vi "Write COM Port.vi"(8 "error in (no error)":errorcluster, 10 "COM Port":refnum<visa-resource-name>, 11 "AirMar in":refnum<class "AirMar.lvclass">) -> (0 "error out":errorcluster, 3 "AirMar out":refnum<class "AirMar.lvclass">)   [LabVIEW 2017, in "Sensors.lvlib" / "AirMar.lvclass"]
uses:
  AirMar.lvclass
  AirMar.lvclass/AirMar.ctl
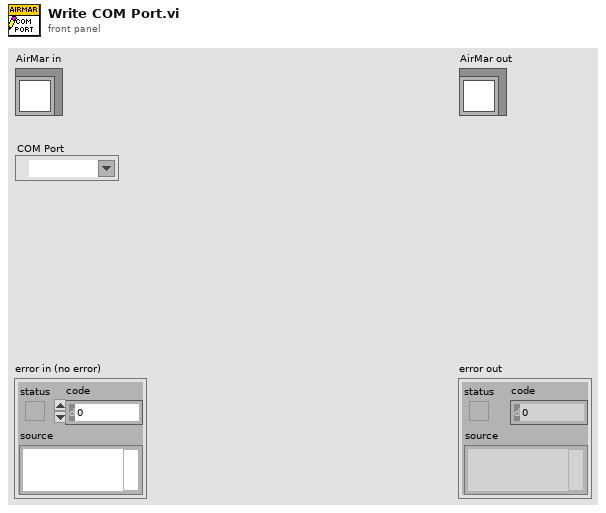
[diagram p1: front panel]
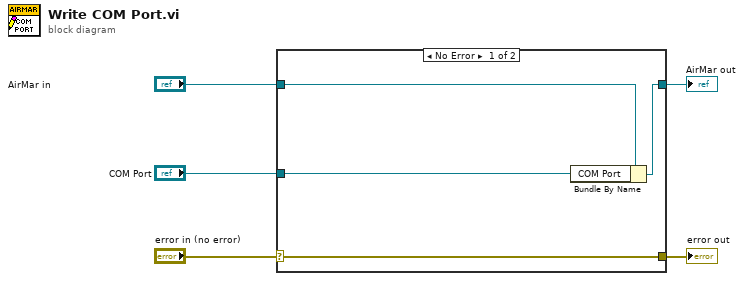
[diagram p0: block diagram]
diagram:
  n1 = case shown="No Error" "error in (no error)" {
    selector: "error in (no error)" -> [w9 w10]
    tunnel: [w9 w10] -> w4
    tunnel: [w7 w11] -> w2
    tunnel: "AirMar in" -> [w8 w11]
    tunnel: "COM Port" -> [w6 _]
    frame No Error {
      n2 = Bundle By Name(cluster=w8, "COM Port"=w6) -> (w7:refnum<class "AirMar.lvclass">)
    }
    frame Error {
    }
  }
  "error out" <- w4
  "AirMar out" <- w2
